vi "CenterFinderSensor_2.vi"(0 "VISA resource name":refnum<visa-resource-name>="COM4", 5 "controller in":refnum<k24>, 9 "Est.Center":T1 {"U" format="%#.5g"; "X" format="%#.5g"; "Y" format="%#.5g"; "Z" format="%#.5g"}, 11 "error in (no error)":errorcluster) -> (4 "VISA resource name out":refnum<visa-resource-name>, 6 "controller out":refnum<k24>, 12 "LaserCenter":T1 {"U" format="%#.5g"; "X" format="%#.5g"; "Y" format="%#.5g"; "Z" format="%#.5g"}, 13 "BoosterCenter":T1 {"U" format="%#.5g"; "X" format="%#.5g"; "Y" format="%#.5g"; "Z" format="%#.5g"}, 14 "NormalCenter":T1 {"U" format="%#.5g"; "X" format="%#.5g"; "Y" format="%#.5g"; "Z" format="%#.5g"}, 15 "error out 2":errorcluster)   [LabVIEW 2016]
uses:
  Control/Coordinate.ctl
  <vilib>/vision/NI_Vision_Development_Module.lvlib
  <vilib>/Instr/_visa.llb/VISA Configure Serial Port (Instr).vi
  <vilib>/Utility/file.llb/Read Delimited Spreadsheet (DBL).vi
  C:/Users/TTUHEP/Documents/LabVIEW/Other Models/2010/Bin/Aerotech.A3200.dll
  Other Models/2010/Bin/Aerotech.A3200.dll
panel:
  out "x/y":dbl
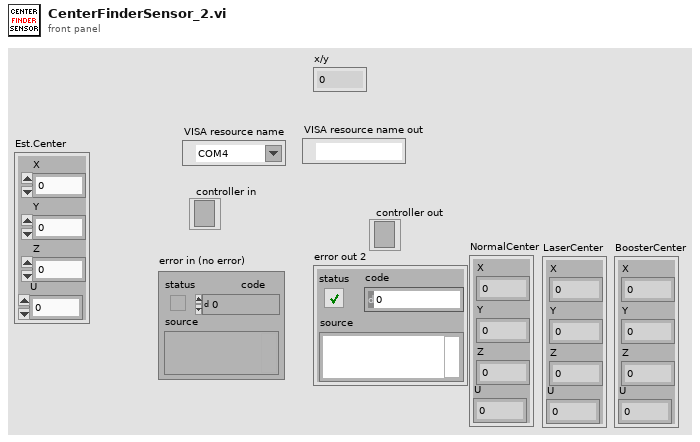
[diagram p1: front panel]
types:
  T1 = typedef "Coordinate.ctl" = cluster{"X":dbl, "Y":dbl, "Z":dbl, "U":dbl}
  T2 = cluster{"Point 1":cluster{"X":sgl, "Y":sgl}, "Point 2":cluster{"X":sgl, "Y":sgl}}
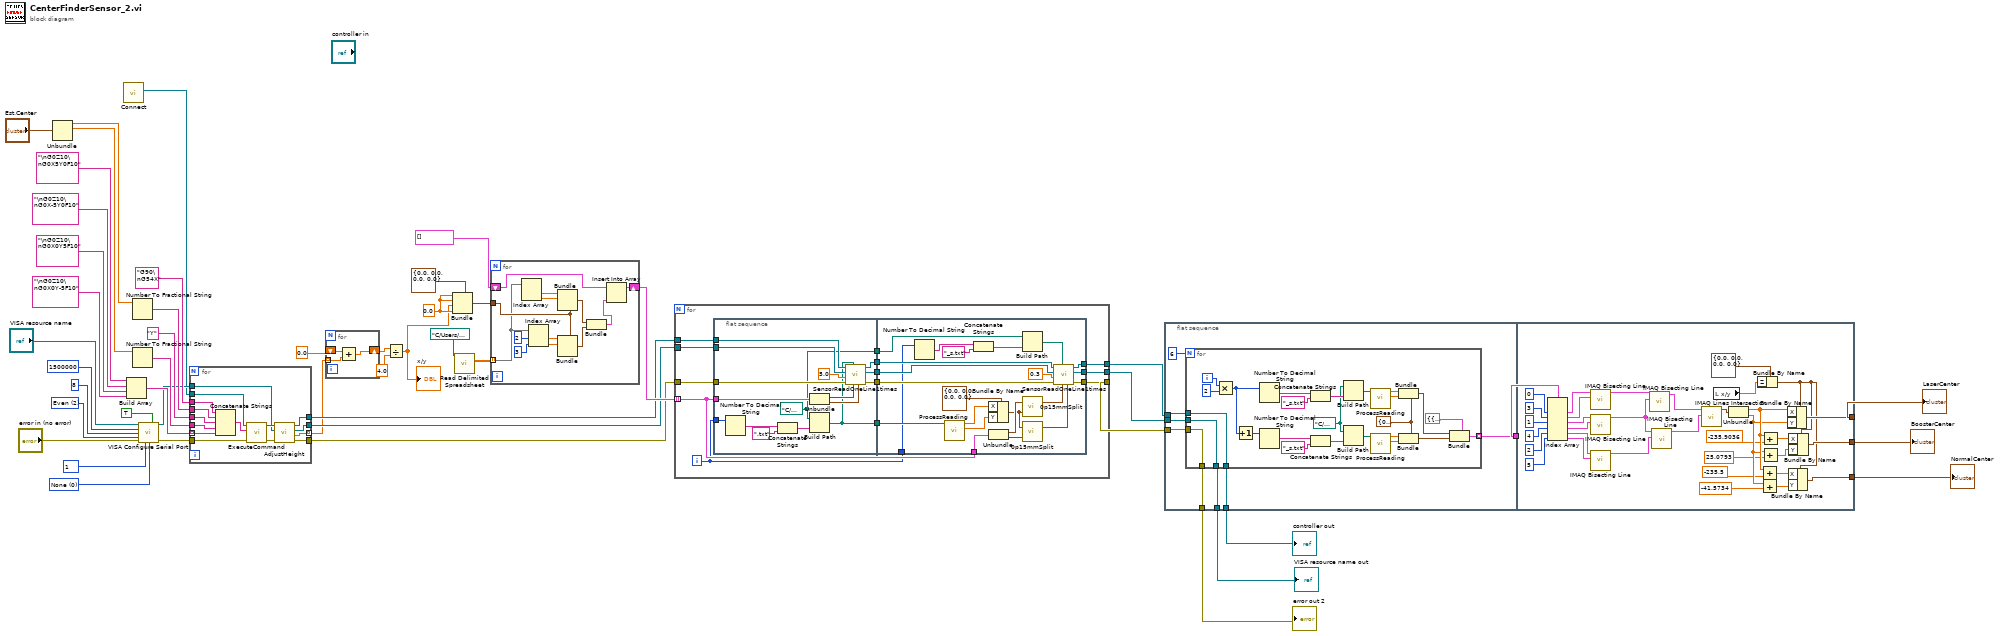
[diagram p0: block diagram]
diagram:
  w37 = u16 0 items=["None"=0, "XON/XOFF"=1, "RTS/CTS"=2, "DTR/DSR"=4] ("flow control")
  w38 = u16 10 items=["1"=10, "1.5"=15, "2.0"=20] ("stop bits")
  w39 = u16 2 items=["None", "Odd", "Even", "Mark", "Space"] ("parity")
  w44 = 0.0
  n1 = Unbundle("Est.Center") -> ("X"=w34:dbl, "Y"=w33:dbl)  [unwired: 2 out]
  n2 = call "Connect.vi"() -> ("controller"=w1:refnum<k24>)  [unwired: 10 in, 1 out]
  n3 = Build Array("\nG0Z10\nG0X5Y0F10", "\nG0Z10\nG0X-5Y0F10", "\nG0Z10\nG0X0Y5F10", "\nG0Z10\nG0X0Y-5F10") -> (w20:string[])
  n4 = Number To Fractional String(number=w34) -> (F-format string=w18:string)  [unwired: 3 in]
  n5 = Number To Fractional String(number=w33) -> (F-format string=w16:string)  [unwired: 3 in]
  n6 = call-poly "VISA Configure Serial Port"("VISA resource name"="VISA resource name", "Enable Termination\nChar (T)"=TRUE, "baud rate (9600)"=u32 1500000 ("baud rate"), "data bits (8)"=u16 8 ("data bits"), "parity (0:none)"=w39, "error in (no error)"="error in (no error)", "stop bits (10: 1 bit)"=w38, "flow control (0:none)"=w37) -> ("VISA resource name out"=w15:refnum<visa-resource-name>, "error out"=w14:errorcluster)  [unwired: 6 in]
  n7 = for {
    tunnel: w20 -> [w63] mode=indexing
    tunnel: "G90\nG54X" -> [w62]
    tunnel: w18 -> [w61]
    tunnel: "Y" -> [w60]
    tunnel: w16 -> [w59]
    tunnel: [w56] -> w10 mode=indexing
    tunnel: [w55] -> w12
    tunnel: [w54] -> w11
    tunnel: w15 -> [w53]
    tunnel: w14 -> [w52]
    tunnel: [w51] -> w13
    tunnel: w1 -> [w50]
    n8 = Concatenate Strings(w62, w61, w60, w59, w63) -> (w49:string)
    n9 = call "ExecuteCommand.vi"("error in (no error)"=w52, "Command Code"=w49, "controller in"=w50) -> ("error out"=w58:errorcluster, "controller out"=w57:refnum<k24>)  [unwired: 6 in, 1 out]
    n10 = call "AdjustHeight.vi"("error in (no error)"=w58, "VISA resource name"=w53, 11:w57) -> ("error out"=w51:errorcluster, "Z Position"=w56:dbl, "VISA resource name out"=w55:refnum<visa-resource-name>, "controller out"=w54:refnum<k24>)  [unwired: 5 in]
  }
  n11 = for {
    tunnel: w10 -> [w64] mode=indexing
    shift-right: [w65] -> w8
    shift-left: 0.0 -> [w66]
    n12 = Add(x=w66, y=w64) -> (x+y=w65:dbl)
  }
  n13 = Divide(x=w8, y=4.0) -> (x/y=w6:dbl)
  "x/y" <- w6
  n14 = Bundle(cluster=T1 {"X"=0.0, "Y"=0.0, "Z"=0.0, "U"=0.0} ("StartPoint"), "X"=w44, "Y"=w44, "Z"=w6, "U"=w44) -> (w43:T1)
  n15 = call-poly <vilib>:"Read Delimited Spreadsheet.vi"("file path (dialog if empty)"=path "C:/Users/TTUHEP/Documents/LabVIEW/Position/CenterTest12Lines.txt") -> ("all rows"=w47:dbl[][])  [unwired: 9 in, 5 out]
  n16 = for {
    tunnel: w47 -> [w78] mode=indexing
    shift-right: [w70] -> w32
    shift-left: cluster{"StartPoint":T1, "StartPoint 2":T1}[] [] -> [w71]
    tunnel: w43 -> [w79]
    n17 = Index Array(array=w78) -> (element #1=w75:dbl, element #2=w74:dbl)  [unwired: 2 in]
    n18 = Index Array(array=w78, index #1=2, index #2=3) -> (element #1=w73:dbl, element #2=w72:dbl)
    n19 = Bundle(cluster=w79, "X"=w75, "Y"=w74) -> (w69:T1)  [unwired: 2 in]
    n20 = Bundle(cluster=w79, "X"=w73, "Y"=w72) -> (w68:T1)  [unwired: 2 in]
    n21 = Bundle("StartPoint"=w69, "StartPoint"=w68) -> (w67:cluster{"StartPoint":T1, "StartPoint":T1})  [unwired: 1 in]
    n22 = Insert Into Array(array=w71, new element=w67) -> (w70:cluster{"StartPoint":T1, "StartPoint 2":T1}[])  [unwired: 1 in]
  }
  n23 = for {
    tunnel: w32 -> [w83] mode=indexing
    tunnel: w11 -> [w90]
    tunnel: w12 -> [w91]
    tunnel: w13 -> [w92]
    tunnel: [w89] -> w30
    tunnel: [w88] -> w31
    tunnel: [w82] -> w29
    i -> [w80]
    n24 = flat-sequence {
      tunnel: w83 -> [w108]
      tunnel: w92 -> [w106]
      tunnel: w91 -> [w105]
      tunnel: w90 -> [w104]
      tunnel: w80 -> [w101]
      tunnel: [w97] -> w87
      tunnel: [w96] -> w86
      tunnel: [w95] -> w85
      tunnel: [w94] -> w84
      tunnel: [w93] -> w81
      tunnel: [w117] -> w88
      tunnel: [w119] -> w89
      tunnel: w87 -> [w122]
      tunnel: w86 -> [w123]
      tunnel: w85 -> [w121]
      tunnel: w84 -> [w131]
      tunnel: w83 -> [w130]
      tunnel: [w118] -> w82
      tunnel: w81 -> [w110]
      tunnel: w80 -> [w114]
      frame #0 {
        w93 = path "C:/Users/TTUHEP/Documents/LabVIEW/Data/Edge"
        n25 = Number To Decimal String(number=w101) -> (decimal integer string=w100:string)  [unwired: 1 in]
        n26 = Concatenate Strings(w100, ".txt") -> (w98:string)
        n27 = Unbundle(w108) -> ("StartPoint"=w107:T1, "StartPoint 2"=w103:T1)
        n28 = Build Path(base path=w93, name or relative path=w98) -> (appended path=w94:path)
        n29 = call "SensorReadOneLine1times.vi"("EndPoint"=w103, "StartPoint"=w107, "file (use dialog)"=w94, "error out"=w106, "Speed"=5.0, "VISA resource name"=w105, "controller"=w104) -> ("error out 2"=w95:errorcluster, "VISA resource name out"=w97:refnum<visa-resource-name>, "controller out"=w96:refnum<k24>)  [unwired: 2 in]
      }
      frame #1 {
        n30 = Number To Decimal String(number=w114) -> (decimal integer string=w113:string)  [unwired: 1 in]
        n31 = call "ProcessReading.vi"("file path (dialog if empty)"=w131) -> ("Y"=w127:dbl, "X"=w128:dbl)  [unwired: 9 in]
        n32 = Concatenate Strings(w113, "_s.txt") -> (w111:string)
        n33 = Unbundle(w130) -> ("StartPoint"=w126:T1, "StartPoint 2"=w124:T1)
        n34 = Bundle By Name(cluster=T1 {"X"=0.0, "Y"=0.0, "Z"=0.0, "U"=0.0} ("StartPoint"), "X"=w128, "Y"=w127) -> (w125:T1)
        n35 = Build Path(base path=w110, name or relative path=w111) -> (appended path=w109:path)
        n36 = call "0p15mmSplit.vi"("EndPoint"=w125, "StartPoint"=w126) -> ("Start"=w116:T1)  [unwired: 1 out]
        n37 = call "0p15mmSplit.vi"("EndPoint"=w124, "StartPoint"=w125) -> ("Start"=w115:T1)  [unwired: 1 out]
        n38 = call "SensorReadOneLine1times.vi"("EndPoint"=w115, "StartPoint"=w116, "file (use dialog)"=w109, "error out"=w121, "Speed"=0.3, "VISA resource name"=w122, "controller"=w123) -> ("error out 2"=w118:errorcluster, "VISA resource name out"=w119:refnum<visa-resource-name>, "controller out"=w117:refnum<k24>)  [unwired: 2 in]
      }
    }
  }
  n39 = flat-sequence {
    tunnel: w31 -> [w137]
    tunnel: w30 -> [w136]
    tunnel: w29 -> [w135]
    tunnel: [w134] -> w27
    tunnel: [w133] -> w26
    tunnel: [w132] -> w25
    tunnel: [w138] -> w5
    tunnel: w5 -> [w181]
    tunnel: [w179] -> w4
    tunnel: [w167] -> w3
    tunnel: [w166] -> w2
    frame #0 {
      n40 = for {
        N: 6 -> [_]
        tunnel: [w143] -> w138 mode=indexing
        tunnel: w137 -> [w141]
        tunnel: w136 -> [w142]
        tunnel: w135 -> [w140]
        tunnel: [w140] -> w132
        tunnel: [w142] -> w133
        tunnel: [w141] -> w134
        i -> [w157]
        w146 = cluster{"X":sgl, "Y":sgl} {"X"=0.0, "Y"=0.0} ("Point 1")
        w154 = path "C:/Users/TTUHEP/Documents/LabVIEW/Data/Edge"
        n41 = Multiply(x=w157, y=2) -> (x*y=w158:i32)
        n42 = Increment(x=w158) -> (x+1=w155:i32)
        n43 = Number To Decimal String(number=w158) -> (decimal integer string=w162:string)  [unwired: 1 in]
        n44 = Number To Decimal String(number=w155) -> (decimal integer string=w160:string)  [unwired: 1 in]
        n45 = Concatenate Strings(w162, "_s.txt") -> (w164:string)
        n46 = Concatenate Strings(w160, "_s.txt") -> (w153:string)
        n47 = Build Path(base path=w154, name or relative path=w164) -> (appended path=w161:path)
        n48 = Build Path(base path=w154, name or relative path=w153) -> (appended path=w152:path)
        n49 = call "ProcessReading.vi"("file path (dialog if empty)"=w161) -> ("Y"=w149:dbl, "X"=w150:dbl)  [unwired: 9 in]
        n50 = call "ProcessReading.vi"("file path (dialog if empty)"=w152) -> ("Y"=w147:dbl, "X"=w148:dbl)  [unwired: 9 in]
        n51 = Bundle(cluster=w146, "X"=w150, "Y"=w149) -> (w145:cluster{"X":sgl, "Y":sgl})
        n52 = Bundle(cluster=w146, "X"=w148, "Y"=w147) -> (w144:cluster{"X":sgl, "Y":sgl})
        n53 = Bundle(cluster=T2 {"Point 1"={"X"=0.0, "Y"=0.0}, "Point 2"={"X"=0.0, "Y"=0.0}} ("Line 1"), "Point 1"=w145, "Point 2"=w144) -> (w143:T2)
      }
    }
    frame #1 {
      n54 = Index Array(array=w181, index #1=0, index #2=3, index #3=1, index #4=4, index #5=2, index #6=5) -> (element #1=w188:T2, element #2=w192:T2, element #3=w193:T2, element #4=w194:T2, element #5=w195:T2, element #6=w189:T2)
      n55 = call "IMAQ Bisecting Line"("Line 2"=w192, "Line 1"=w188) -> ("Bisecting Line"=w196:T2)  [unwired: 8 in, 1 out]
      n56 = call "IMAQ Bisecting Line"("Line 2"=w194, "Line 1"=w193) -> ("Bisecting Line"=w197:T2)  [unwired: 8 in, 1 out]
      n57 = call "IMAQ Bisecting Line"("Line 2"=w189, "Line 1"=w195) -> ("Bisecting Line"=w198:T2)  [unwired: 8 in, 1 out]
      n58 = call "IMAQ Bisecting Line"("Line 2"=w197, "Line 1"=w196) -> ("Bisecting Line"=w190:T2)  [unwired: 8 in, 1 out]
      n59 = call "IMAQ Bisecting Line"("Line 2"=w198, "Line 1"=w197) -> ("Bisecting Line"=w191:T2)  [unwired: 8 in, 1 out]
      n60 = call "IMAQ Lines Intersection"("Line 2"=w191, "Line 1"=w190) -> ("Intersection Point"=w199:cluster{"X":sgl, "Y":sgl})  [unwired: 7 in, 2 out]
      n61 = local read "x/y"() -> (w180:dbl)
      n62 = Unbundle(w199) -> ("X"=w173:sgl, "Y"=w172:sgl)
      n63 = Bundle By Name(cluster=T1 {"X"=0.0, "Y"=0.0, "Z"=0.0, "U"=0.0} ("Est.Center 2"), "Z"=w180) -> (w165:T1)
      n64 = Add(x=w173, y=-235.5) -> (x+y=w175:dbl)
      n65 = Add(x=w172, y=-41.5734) -> (x+y=w174:dbl)
      n66 = Add(x=w173, y=-235.9036) -> (x+y=w177:dbl)
      n67 = Add(x=w172, y=25.0793) -> (x+y=w176:dbl)
      n68 = Bundle By Name(cluster=w165, "X"=w173, "Y"=w172) -> (w179:T1)
      n69 = Bundle By Name(cluster=w165, "X"=w175, "Y"=w174) -> (w166:T1)
      n70 = Bundle By Name(cluster=w165, "X"=w177, "Y"=w176) -> (w167:T1)
    }
  }
  "controller out" <- w27
  "VISA resource name out" <- w26
  "error out 2" <- w25
  "LaserCenter" <- w4
  "BoosterCenter" <- w3
  "NormalCenter" <- w2
